vi "LEP_RV_Timer_Config.vi"(8 "error in (no error)":errorcluster, 10 "Config Data":string[](array[string]), 11 "Interrupt Name":string) -> (0 "error out":errorcluster, 3 "Interrupt Configuration":string[](array[string]))   [LabVIEW 2011]
panel:
  in  "help":bool
  in  "Units":u16(ring)=1 items=["Ticks", "Milliseconds"]
  in  "cancel":bool
  in  "ok":bool
  in  "Period":i32=1000
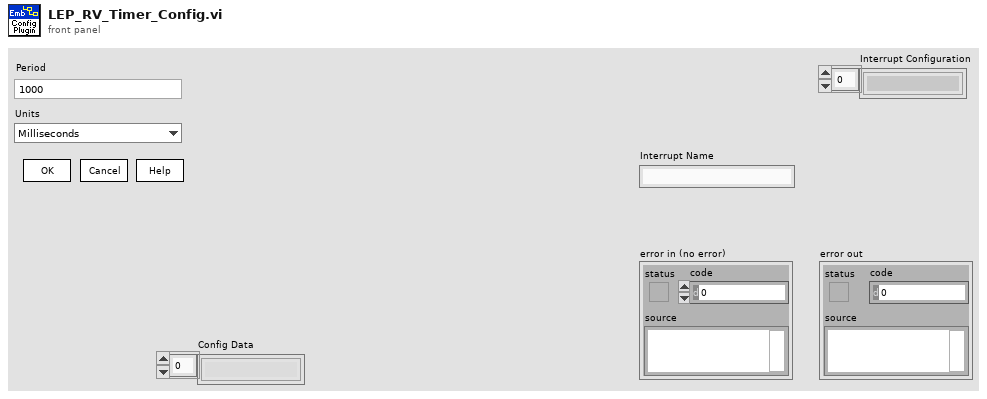
[diagram p1: front panel]
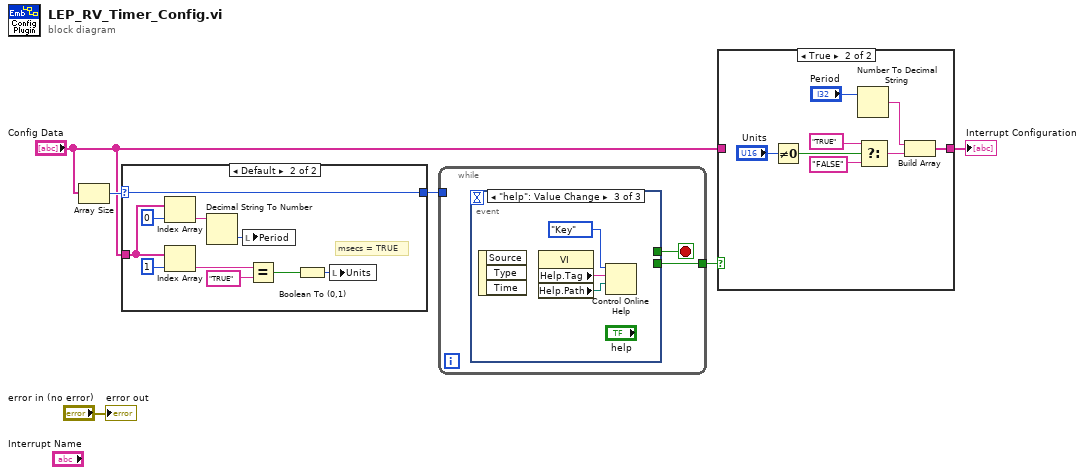
[diagram p0: block diagram]
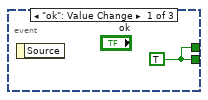
[diagram p4: hidden frame]
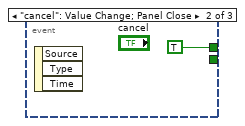
[diagram p5: hidden frame]
diagram:
  n1 = Array Size(array="Config Data") -> (size(s)=w2:i32)
  n2 = case shown="Default" w2 {
    selector: w2 -> [w7 w14]
    tunnel: [w7 w14] -> w4
    tunnel: "Config Data" -> [_ w8]
    frame 0 {
    }
    frame Default {
      # "msecs = TRUE"
      n3 = Index Array(array=w8, index=0) -> (element=w10:string)
      n4 = Index Array(array=w8, index=1) -> (element=w11:string)
      n5 = Decimal String To Number(string=w10) -> (number=w9:i32)  [unwired: 3 out]
      n6 = local write "Period"(w9) -> ()
      n7 = Equal?(x=w11, y="TRUE") -> (x = y?=w16:bool)
      n8 = Boolean To (0,1)(Boolean=w16) -> (0, 1=w15:i16)
      n9 = local write "Units"(w15) -> ()
    }
  }
  n10 = while {
    tunnel: [w18] -> w5
    tunnel: w4 -> [_]
    stop <- w19 stop-if-true
    n11 = event shown="[2] \"help\": Value Change" {
      selector: _ -> [_ _ _]
      dyn-events: _ -> [_ _ _]
      timeout: _ -> [_ _ _]
      tunnel: [w20 TRUE _] -> w19
      tunnel: [w20 _ _] -> w18
      event "ok": Value Change {
        w20 = TRUE
        n12 = event-data() -> ()  [unwired: 2 out]
      }
      event "cancel": Value Change; Panel Close {
        n13 = event-data() -> ()  [unwired: 4 out]
      }
      event "help": Value Change {
        n14 = event-data() -> ()  [unwired: 4 out]
        n15 = property class="VI"() -> ("Help.Tag"=w23:string, "Help.Path"=w24:path)  [unwired: 2 in, 2 out]
        n16 = Control Online Help(2:w24, 3:w23, 4:enum16{"Contents", "Key", "Close"}."Key" ("Operation")) -> ()  [unwired: 1 in, 1 out]
      }
    }
  }
  n17 = case shown="True" w5 {
    tunnel: [w25 w26] -> w3
    tunnel: "Config Data" -> [w25 _]
    frame False {
    }
    frame True {
      n18 = Not Equal To 0?(x="Units") -> (x != 0?=w32:bool)
      n19 = Number To Decimal String(number="Period") -> (decimal integer string=w27:string)  [unwired: 1 out]
      n20 = Select(t="TRUE", s=w32, f="FALSE") -> (s? t:f=w28:string)
      n21 = Build Array(w27, w28) -> (w26:string[])
    }
  }
  "Interrupt Configuration" <- w3
  "error out" <- "error in (no error)"
